vi "Manual Control.vi"(8 "error in (no error)":errorcluster) -> (0 "error out":errorcluster)   [LabVIEW 2012, in "Stepper.lvclass"]
uses:
  Stepper.lvclass
  Stepper.lvclass/Stepper.ctl
panel:
  out "Position":i32(slide) scale=0.0..100.0
  in  "endprgm":bool
  in  "Start/Stop":bool
  in  "Speed":dbl[unit]=5e-09
  in  "Direction":bool
  out "Coil Status":bool[](array[boolean])=[TRUE, TRUE, TRUE, TRUE, TRUE, TRUE, TRUE, TRUE]
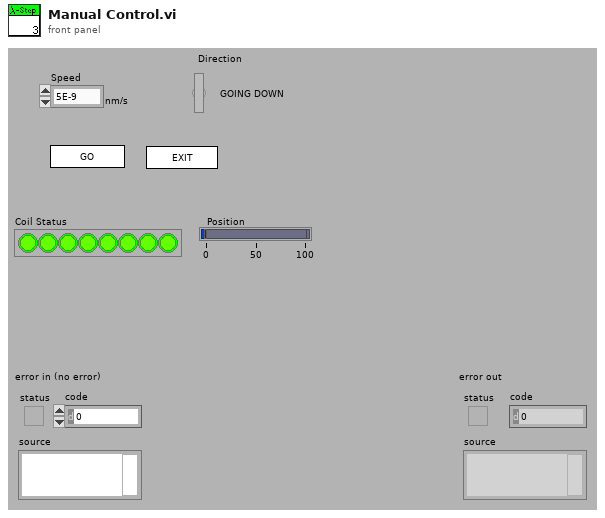
[diagram p1: front panel]
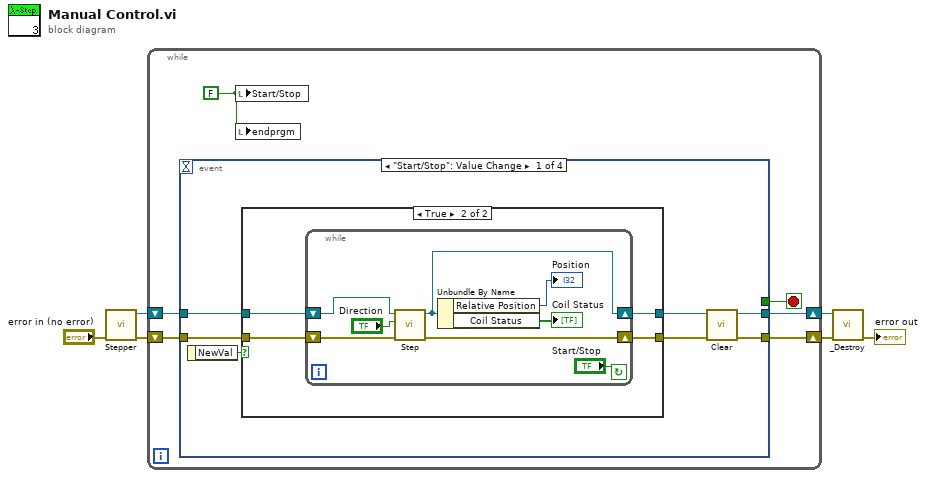
[diagram p0: block diagram]
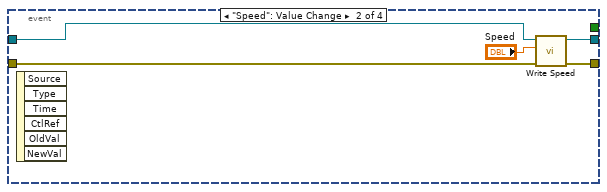
[diagram p3: hidden frame]
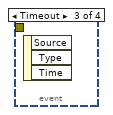
[diagram p4: hidden frame]
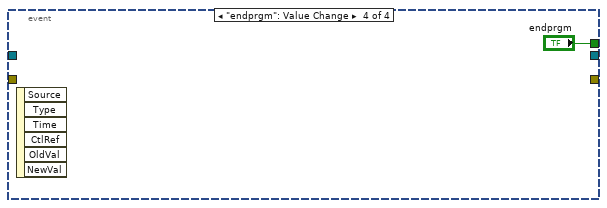
[diagram p5: hidden frame]
diagram:
  n1 = call "Stepper.vi"("error in (no error)"="error in (no error)") -> ("error out"=w3:errorcluster, "Stepper out"=w2:refnum<class "Stepper.lvclass">)  [unwired: 9 out]
  n2 = while {
    shift-right: [w10] -> w4
    shift-left: w2 -> [w7]
    shift-right: [w8] -> w1
    shift-left: w3 -> [w9]
    stop <- w12 stop-if-true
    w11 = FALSE
    n3 = event shown="[0] \"Start/Stop\": Value Change" {
      selector: _ -> [_ _ _ _]
      dyn-events: _ -> [_ _ _ _]
      timeout: _ -> [_ _ _ _]
      tunnel: [_ _ _ "endprgm"] -> w12
      tunnel: [w13 w37 _ _] -> w10
      tunnel: w7 -> [w18 w36 _ _]
      tunnel: w9 -> [w17 w35 _ _]
      tunnel: [w15 w34 _ _] -> w8
      event "Start/Stop": Value Change {
        n4 = event-data() -> ("NewVal"=w19:bool)  [unwired: 1 out]
        n5 = case shown="True" w19 {
          tunnel: [w21 w25] -> w14
          tunnel: w18 -> [w21 w24]
          tunnel: w17 -> [w20 w23]
          tunnel: [w20 w22] -> w16
          frame False {
          }
          frame True {
            n6 = while {
              shift-right: [w28] -> w25
              shift-left: w24 -> [w29]
              shift-right: [w32] -> w22
              shift-left: w23 -> [w30]
              stop <- "Start/Stop" continue-if-true
              n7 = call "Step.vi"("error in"=w30, "Up?"="Direction", "Stepper.lvclass"=w29) -> ("error out"=w32:errorcluster, "Stepper.lvclass out"=w28:refnum<class "Stepper.lvclass">)  [unwired: 1 in, 6 out]
              n8 = Unbundle By Name(w28) -> ("Relative Position"=→"Position":i32, "Coil Status"=→"Coil Status":bool[])
            }
          }
        }
        n9 = call-dynamic "Clear.vi"("error in (no error)"=w16, "Stepper in"=w14) -> ("error out"=w15:errorcluster, "Stepper out"=w13:refnum<class "Stepper.lvclass">)  [unwired: 8 out]
      }
      event "Speed": Value Change {
        n10 = event-data() -> ()  [unwired: 7 out]
        n11 = call-dynamic "Write Speed.vi"("error in (no error)"=w35, "Speed"="Speed", "Stepper.lvclass in"=w36) -> ("error out"=w34:errorcluster, "Stepper.lvclass out"=w37:refnum<class "Stepper.lvclass">)  [unwired: 7 out]
      }
      event Timeout {
        n12 = event-data() -> ()  [unwired: 4 out]
      }
      event "endprgm": Value Change {
        n13 = event-data() -> ()  [unwired: 7 out]
      }
    }
    n14 = local write "Start/Stop"(w11) -> ()
    n15 = local write "endprgm"(w11) -> ()
  }
  n16 = call-dynamic "_Destroy.vi"("error in (no error)"=w1, "Stepper in"=w4) -> ("error out"=→"error out":errorcluster)  [unwired: 9 out]
